vi "PlayCancelEnabler.vi"(8 "error in (no error)":errorcluster, 10 "Game in progress?":bool, 11 "General Refs":T1) -> (0 "error out":errorcluster)   [LabVIEW 2020]
uses:
  controls/General Refnums.ctl
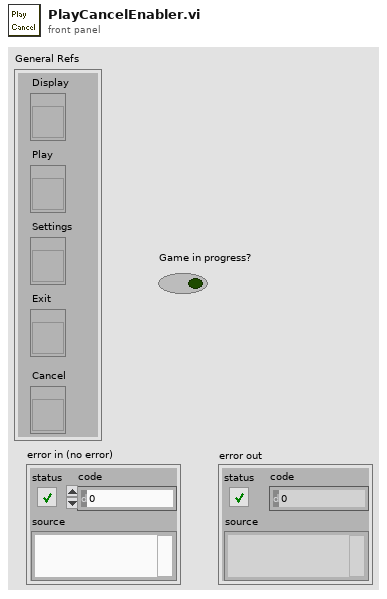
[diagram p1: front panel]
types:
  T1 = typedef "General Refnums.ctl" = cluster{"Display":refnum<vi>, "Play":refnum<vi>, "Settings":refnum<vi>, "Exit":refnum<vi>, "Cancel":refnum<vi>}
  T2 = enum8{"Enabled", "Disabled", "Disabled and Grayed Out"}
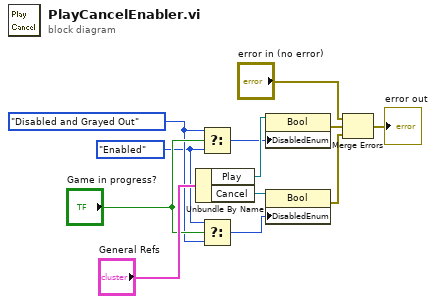
[diagram p0: block diagram]
diagram:
  w2 = T2."Disabled and Grayed Out" ("Disabled")
  w1 = T2."Enabled" ("Disabled")
  n1 = Unbundle By Name("General Refs") -> ("Play"=w11:refnum<vi>, "Cancel"=w10:refnum<vi>)
  n2 = Select(t=w2, s="Game in progress?", f=w1) -> (s? t:f=w5:T2)
  n3 = Select(t=w1, s="Game in progress?", f=w2) -> (s? t:f=w4:T2)
  n4 = property on="Property Node" class="Bool"(reference=w11, "DisabledEnum"=w5) -> (error out=w7:errorcluster)  [unwired: 1 in, 1 out]
  n5 = property on="Property Node" class="Bool"(reference=w10, "DisabledEnum"=w4) -> (error out=w6:errorcluster)  [unwired: 1 in, 1 out]
  n6 = Merge Errors("error in (no error)", w7, w6) -> (→"error out":errorcluster)
